vi "Simple Mapping.vi"() -> ()   [LabVIEW 2009]
uses:
  <vilib>/Platform/TimedLoop/XDataNode/XDataNode.xnode
  <vilib>/Platform/TimedLoop/XDataNode/loadlvalarms.vi
  <vilib>/Platform/TimedLoop/XDataNode/timing_clust.ctl
  <vilib>/Platform/TimedLoop/XDataNode/nitl_modes.ctl
  <vilib>/Platform/TimedLoop/XDataNode/wakeup.ctl
  <vilib>/Platform/TimedLoop/XDataNode/XDNodeRunTimeDep.lvlib
panel:
  out "XY Graph 2":cluster{"Y":dbl[], "Y":dbl[]}[](graph)
  in  "stop":bool
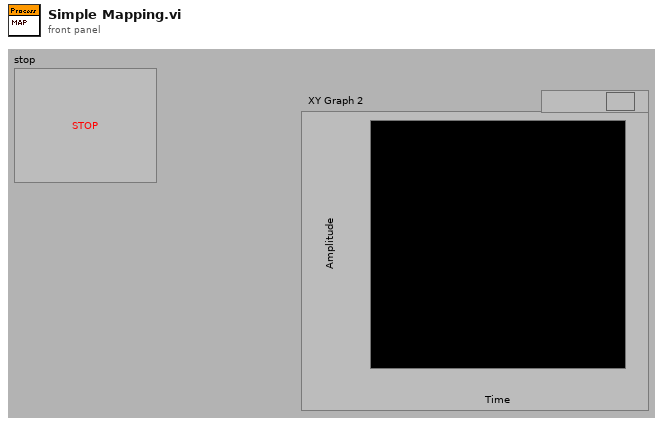
[diagram p1: front panel]
types:
  T1 = typedef "XDNodeRunTimeDep.lvlib/timing_clust.ctl" = cluster{"Expected End [f-1]":u64, "Actual End [f-1]":u64, "Finished Late? [f-1]":bool, "Expected End [i-1]":u64, "Actual End [i-1]":u64, "Finished Late? [i-1]":bool, "Expected Start [i]":u64, "Actual Start [i]":u64, "Expected Start [f]":u64, "Actual Start [f]":u64, "Source Name":string, "Structure Name":string, "Period":i64, "Deadline":i64, "Offset":i64, "Start":i64, "Priority":i32, "Timeout":i32, "Mode":T2, "Wakeup Reason":T3, "Error":errorcluster, "Source Type":string, "Secondary Source Type":string, "Global End Time":u64, "Global Start Time":u64, "Frame Duration":u64, "Iteration Duration":u64, "Assigned CPU":i32, "I/O Scan Engine Mode":u32}
  T2 = typedef "XDNodeRunTimeDep.lvlib/nitl_modes.ctl" = enum32{"No Change", "Process missed periods, maintain original phase", "Discard missed periods, maintain original phase", "Process missed periods, ignore original phase", "Discard missed periods, ignore original phase"}
  T3 = typedef "XDNodeRunTimeDep.lvlib/wakeup.ctl" = enum32{"Normal", "Aborted", "Asynchronous wakeup", "Timing source error", "Timed loop error", "Timeout"}
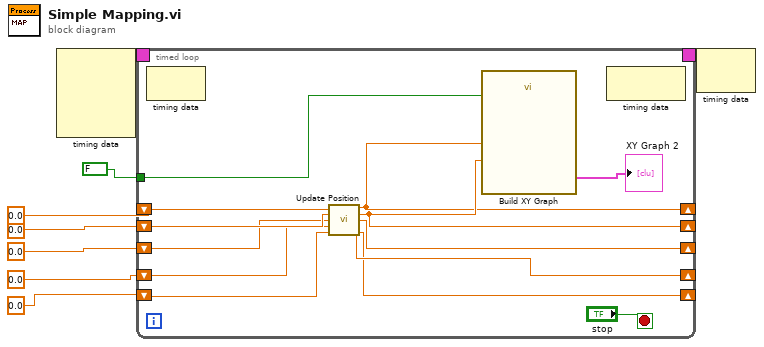
[diagram p0: block diagram]
diagram:
  n1 = node-c288() -> (w5:T1)  [unwired: 4 in]
  n2 = timed-loop {
    shift-right: [w17] -> _
    shift-left: 0.0 ("Last Position X") -> [w15]
    shift-right: [w18] -> _
    shift-left: 0.0 ("Last Position X") -> [w14]
    shift-right: [w21] -> _
    shift-left: 0.0 ("Last Position X") -> [w13]
    timing: w5 -> [_]
    timing-out: [_] -> w4
    tunnel: FALSE -> [w16]
    shift-right: [w10] -> _
    shift-left: 0.0 ("Last Position X") -> [w12]
    shift-right: [w9] -> _
    shift-left: 0.0 ("Last Position X") -> [w11]
    stop <- "stop" stop-if-true
    n3 = node-c288() -> ()  [unwired: 1 in, 1 out]
    n4 = call "Update Position.vi"("Last Position X"=w15, "Last Postion Y"=w14, "Last Postion Z"=w13, "Last Left Dist"=w12, "Last Right Dist"=w11) -> ("New X"=w17:dbl, "New Y"=w18:dbl, "New Z"=w21:dbl, "Left Dist Travelled Out (cm)"=w10:dbl, "Right Dist Travelled Out (cm)"=w9:dbl)  [unwired: 6 in]
    n5 = call "Build XY Graph"("Reset"=w16, "Y Input"=w18, "X Input"=w17) -> ("XY Graph"=→"XY Graph 2":cluster{"Y":dbl[], "Y":dbl[]}[])  [unwired: 7 in, 1 out]
    n6 = node-c288() -> ()  [unwired: 1 in, 1 out]
  }
  n7 = node-c288(w4) -> ()  [unwired: 1 out]
